vi "exercise2_firstvi_subvi.vi"(11 "angulo grados":dbl) -> (3 "coseno(angulo)":dbl(knob) scale=0.0..1.0)   [LabVIEW 2018]
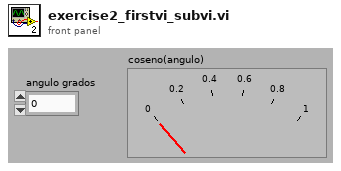
[diagram p1: front panel]
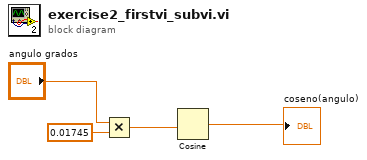
[diagram p0: block diagram]
diagram:
  n1 = Multiply(x="angulo grados", y=0.01745) -> (x*y=w1:dbl)
  n2 = Cosine(x=w1) -> (cos(x)=→"coseno(angulo)":dbl)
